vi "Destroy User Event - Stop.vi"(8 "error in (no error)":T1 caption="entrée d'erreur (pas d'erreur)", 11 "Événement utilisateur - Arrêt":refnum<user-event>) -> (0 "error out":T1 caption="sortie d'erreur")   [LabVIEW 2020, in "User Event - Stop.lvlib"]
doc: "Supprimer l'événement utilisateur, même s'il y a une erreur en entrée."
uses:
  User Event - Stop.lvlib
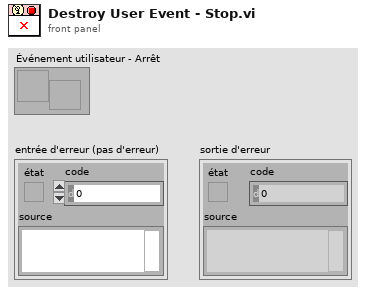
[diagram p1: front panel]
types:
  T1 = cluster{"état":bool, "code":i32, "source":string}
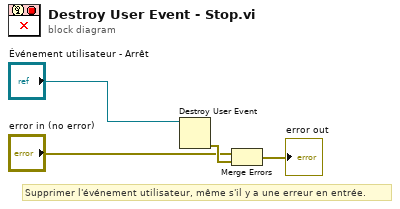
[diagram p0: block diagram]
diagram:
  # "Supprimer l'événement utilisateur, même s'il y a une erreur en entrée."
  n1 = Destroy User Event(user event="Événement utilisateur - Arrêt") -> (error out=w3:errorcluster)  [unwired: 1 in]
  n2 = Merge Errors("error in (no error)", w3) -> (→"error out":errorcluster)
